vi "Extract_2D_Array.vi"() -> ()   [LabVIEW 2020]
panel:
  out "THIRD_ROW":dbl[](graph)
  out "SECOND_ROW":dbl[](graph)
  out "FIRST_ROW":dbl[](graph)
  out "Random_Matrix":dbl[][](array[numeric])
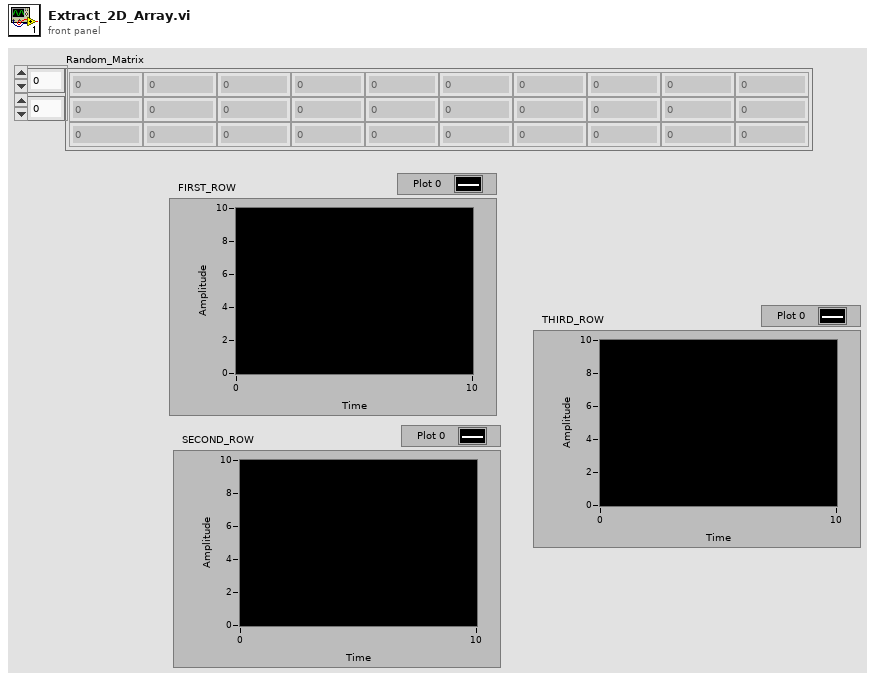
[diagram p1: front panel]
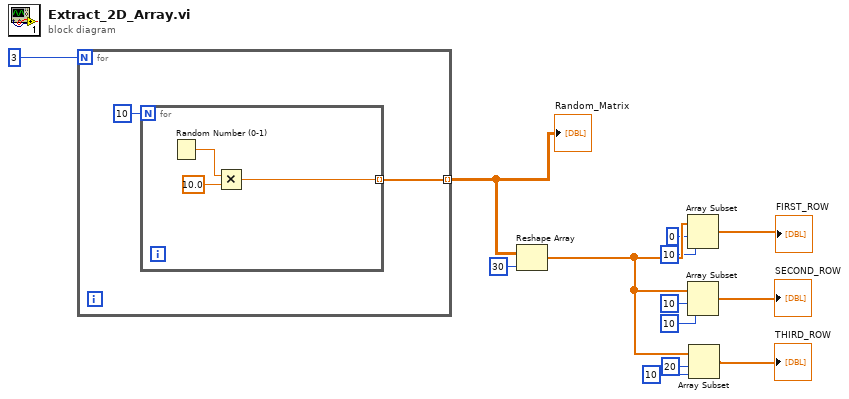
[diagram p0: block diagram]
diagram:
  n1 = for {
    N: 3 -> [_]
    tunnel: [w14] -> w12 mode=indexing
    n2 = for {
      N: 10 -> [_]
      tunnel: [w16] -> w14 mode=indexing
      n3 = Random Number (0-1)() -> (number: 0 to 1=w18:dbl)
      n4 = Multiply(x=w18, y=10.0) -> (x*y=w16:dbl)
    }
  }
  "Random_Matrix" <- w12
  n5 = Reshape Array(w12, 30 ("dimension size")) -> (w10:dbl[])
  n6 = Array Subset(array=w10, index=0, length=10) -> (→"FIRST_ROW":dbl[])
  n7 = Array Subset(array=w10, index=10, length=10) -> (→"SECOND_ROW":dbl[])
  n8 = Array Subset(array=w10, index=20, length=10) -> (→"THIRD_ROW":dbl[])
